vi "Set Data to print.vi"(8 "error in (no error)":errorcluster caption="entrée d'erreur (pas d'erreur)", 10 "Data to print":string, 11 "Class Printer (Default) en entrée":refnum<class "Class Printer (Default).lvclass">) -> (0 "error out":errorcluster caption="sortie d'erreur", 3 "Class Printer (Default) en sortie":refnum<class "Class Printer (Default).lvclass">)   [LabVIEW 2020, in "Library Instrument & Equipement.lvlib" / "Library Printer.lvlib" / "Class Printer (Default).lvclass"]
uses:
  Class Printer (Default).lvclass
  Class Printer (Default).lvclass/Class Printer (Default).ctl
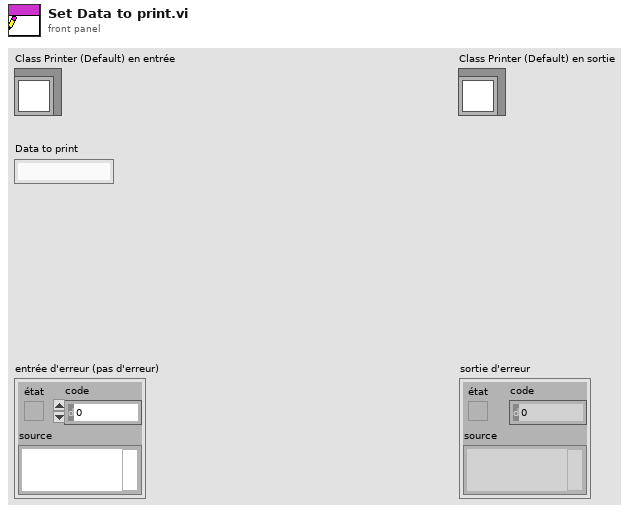
[diagram p1: front panel]
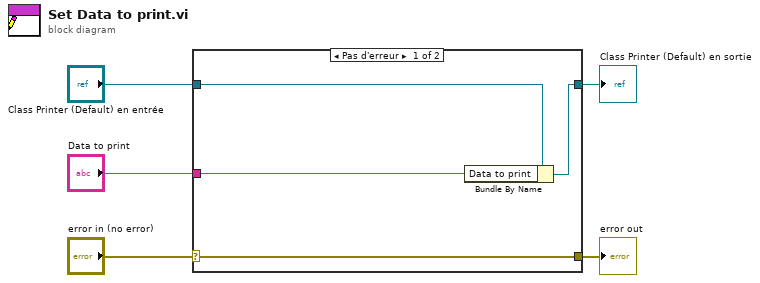
[diagram p0: block diagram]
diagram:
  n1 = case shown="Pas d'erreur" "error in (no error)" {
    selector: "error in (no error)" -> [w9 w10]
    tunnel: [w9 w10] -> w4
    tunnel: [w7 w11] -> w2
    tunnel: "Class Printer (Default) en entrée" -> [w8 w11]
    tunnel: "Data to print" -> [w6 _]
    frame No Error {
      n2 = Bundle By Name(cluster=w8, "Data to print"=w6) -> (w7:refnum<class "Class Printer (Default).lvclass">)
    }
    frame Error {
    }
  }
  "error out" <- w4
  "Class Printer (Default) en sortie" <- w2
